vi "HMI_OpenFileDialog.vi"(10 "Root Name":string="PWC-OLS", 11 "relative path":path=path "$ReportFiles") -> (0 "selected path":path, 1 "File Name":string, 2 "Root Path":path)   [LabVIEW 2024]
doc: "Use to create relative paths to make the program portable.I\n\niNPUTS\nRelative Path is the name of the folder where to begin the file open dialog.\nRoot Name is the String name of the Root folder of this program.\n\nOUTPUS\nFile Path Path to the Opened File\nRoot Path Path to the root Folder\nFile Name String name less Path and extension."
uses:
  <vilib>/regexp/Match Regular Expression.xnode
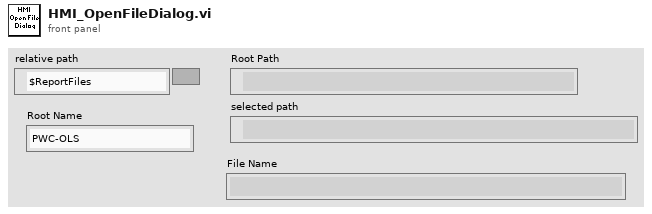
[diagram p1: front panel]
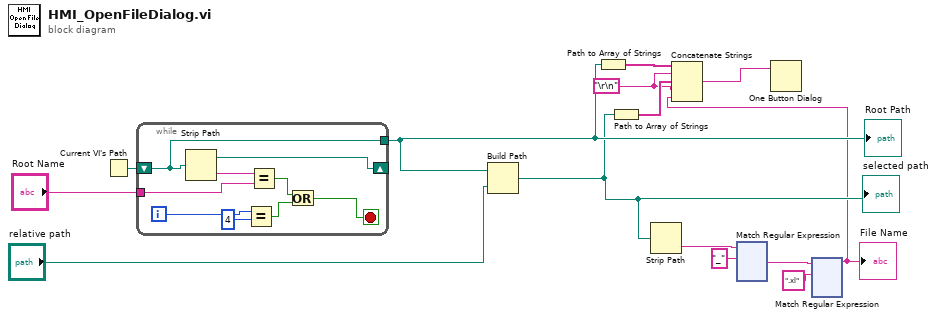
[diagram p0: block diagram]
diagram:
  w3 = "\r\n"
  n1 = Current VI's Path() -> (path=w14:path)
  n2 = while {
    shift-right: [w17] -> _
    shift-left: w14 -> [w16]
    tunnel: [w16] -> w7
    tunnel: "Root Name" -> [w15]
    i -> [w22]
    stop <- w18 stop-if-true
    n3 = Strip Path(path=w16) -> (stripped path=w17:path, name=w23:string)
    n4 = Equal?(x=w22, y=4) -> (x = y?=w19:bool)
    n5 = Equal?(x=w23, y=w15) -> (x = y?=w20:bool)
    n6 = Or(x=w20, y=w19) -> (x .or. y?=w18:bool)
  }
  "Root Path" <- w7
  n7 = Build Path(base path=w7, name or relative path="relative path") -> (appended path=w4:path)
  "selected path" <- w4
  n8 = Path to Array of Strings(0:w7) -> (2:w6:string[])  [unwired: 1 out]
  n9 = Path to Array of Strings(0:w4) -> (2:w5:string[])  [unwired: 1 out]
  n10 = Strip Path(path=w4) -> (name=w10:string)  [unwired: 1 out]
  n11 = xnode "Match Regular Expression"("input string"=w10, "regular expression"="_") -> ("after match"=w9:string)  [unwired: 4 in, 4 out]
  n12 = xnode "Match Regular Expression"("input string"=w9, "regular expression"=".xl") -> ("before match"=w2:string)  [unwired: 4 in, 4 out]
  "File Name" <- w2
  n13 = Concatenate Strings(w6, w3, w5, w3, w2) -> (w1:string)
  n14 = One Button Dialog(message=w1) -> ()  [unwired: 1 in, 1 out]
